vi "Copy lvlib To Disk.vi"(6 "Created Library File Path":path, 8 "error in":errorcluster, 9 "Template Library File Path":path, 10 "NI.LV.Dialog Instance":refnum<vi>) -> (0 "error out":errorcluster)   [LabVIEW 2020, in "_Template.lvlib" / "_Template.lvclass"]
uses:
  _Template.lvclass
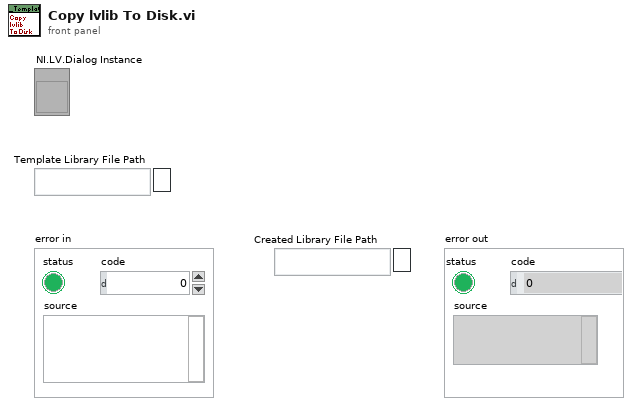
[diagram p1: front panel]
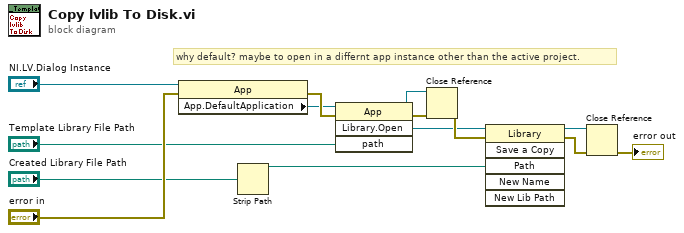
[diagram p0: block diagram]
diagram:
  # "why default? maybe to open in a differnt app instance other than the active project."
  n1 = property class="App"(reference="NI.LV.Dialog Instance", error in="error in") -> (error out=w13:errorcluster, "App.DefaultApplication"=w9:refnum<vi>)  [unwired: 1 out]
  n2 = Strip Path(path="Created Library File Path") -> (stripped path=w1:path)  [unwired: 1 out]
  n3 = invoke class="App" method="Library.Open"(reference=w9, error in=w13, "path"="Template Library File Path") -> (reference out=w8:refnum<vi>, error out=w14:errorcluster, "Open Library"=w11:refnum<vi>)  [unwired: 1 in, 1 out]
  n4 = Close Reference(reference=w8, error in (no error)=w14) -> (error out=w12:errorcluster)
  n5 = invoke class="Library" method="Save a Copy"(reference=w11, error in=w12, "Path"=w1) -> (reference out=w10:refnum<vi>, error out=w7:errorcluster)  [unwired: 3 in, 4 out]
  n6 = Close Reference(reference=w10, error in (no error)=w7) -> (error out=→"error out":errorcluster)
